vi "MQTT_Q_Publish.vi"(6 "Topic":string, 8 "error in":errorcluster, 10 "Message":string, 11 "MQTT_Q In":refnum<class "MQTT_Q.lvclass">) -> (0 "error out":errorcluster, 3 "MQTT_Q Out":refnum<class "MQTT_Q.lvclass">)   [LabVIEW 2015, in "MQTT_Q.lvclass"]
uses:
  MQTT_Q.lvclass
  MQTT_Q_PVT_MessageType.ctl
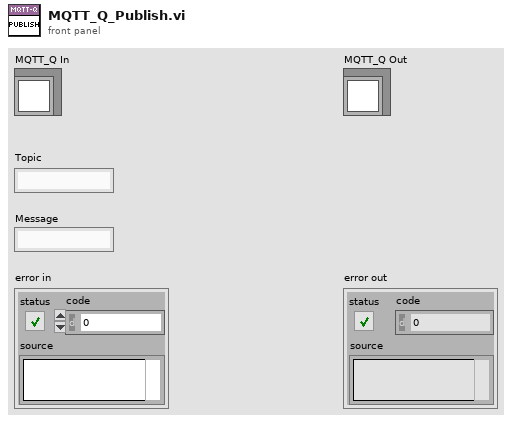
[diagram p1: front panel]
types:
  T1 = typedef "MQTT_Q.lvclass/MQTT_Q_PVT_MessageType.ctl" = enum32{"Reserved", "CONNECT", "CONNACK", "PUBLISH", "PUBACK", "PUBREC", "PUBREL", "PUBCOMP", "SUBSCRIBE", "SUBACK", "UNSUBSCRIBE", "UNSUBACK", "PINGREQ", "PINGRESP", "DISCONNECT", "Reserved2"}
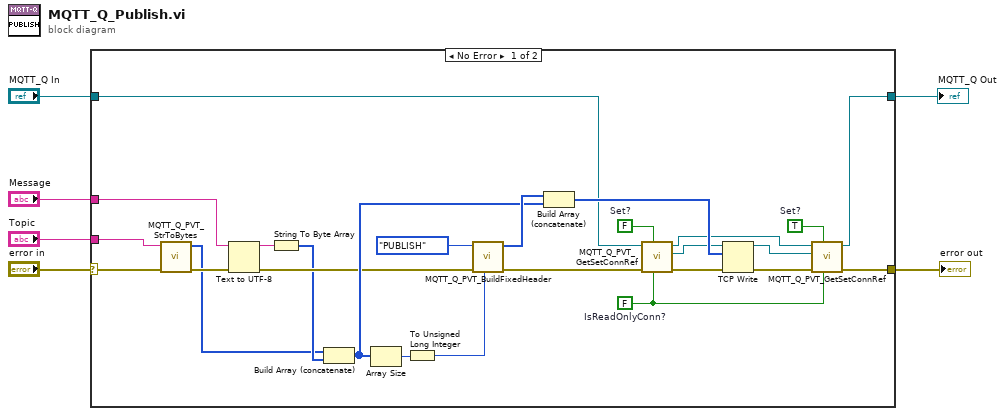
[diagram p0: block diagram]
diagram:
  n1 = case shown="No Error" "error in" {
    selector: "error in" -> [w22 w34]
    tunnel: [w16 w34] -> w5
    tunnel: "MQTT_Q In" -> [w14 w33]
    tunnel: [w13 w33] -> w3
    tunnel: "Topic" -> [w8 _]
    tunnel: "Message" -> [w9 _]
    frame No Error {
      w10 = FALSE  # IsReadOnlyConn?
      w20 = FALSE  # Set?
      w21 = TRUE  # Set?
      n2 = call "MQTT_Q_PVT_StrToBytes.vi"("error in (no error)"=w22, "String in"=w8) -> ("error out"=w23:errorcluster, "Bytes out"=w7:u8[])  [unwired: 8 in]
      n3 = Text to UTF-8(8:w23, 11:w9) -> (0:w25:errorcluster, 3:w26:string)  [unwired: 1 in]
      n4 = String To Byte Array(string=w26) -> (unsigned byte array=w24:u8[])
      n5 = Build Array (concatenate)(w7, w24) -> (w28:u8[])
      n6 = Array Size(array=w28) -> (size(s)=w30:i32)
      n7 = To Unsigned Long Integer(number=w30) -> (unsigned 32bit integer=w31:u32)
      n8 = call "MQTT_Q_PVT_BuildFixedHeader.vi"("Remaining Length"=w31, "error in (no error)"=w25, "MessageType"=MQTT_Q_PVT_MessageType."PUBLISH") -> ("error out"=w19:errorcluster, "Fixed Header"=w29:u8[])  [unwired: 7 in]
      n9 = Build Array (concatenate)(w29, w28) -> (w27:u8[])
      n10 = call "MQTT_Q_PVT_GetSetConnRef.vi"("IsReadOnlyConn?"=w10, "Set?"=w20, "error in (no error)"=w19, "MQTT_Q in"=w14) -> ("error out"=w18:errorcluster, "connection ID Out"=w12:refnum<k5>, "MQTT_Q out"=w15:refnum<class "MQTT_Q.lvclass">)  [unwired: 5 in]
      n11 = TCP Write(connection ID=w12, data in=w27, error in (no error)=w18) -> (connection ID out=w11:refnum<k5>, error out=w17:errorcluster)  [unwired: 1 in, 1 out]
      n12 = call "MQTT_Q_PVT_GetSetConnRef.vi"("IsReadOnlyConn?"=w10, "Set?"=w21, "error in (no error)"=w17, "connection ID In"=w11, "MQTT_Q in"=w15) -> ("error out"=w16:errorcluster, "MQTT_Q out"=w13:refnum<class "MQTT_Q.lvclass">)  [unwired: 4 in, 1 out]
    }
    frame Error {
    }
  }
  "error out" <- w5
  "MQTT_Q Out" <- w3
